vi "Software Update HCC Search For Archive.vi"(8 "error in (no error)":errorcluster, 10 "folder names":string[](array[string]), 11 "Path":path) -> (0 "error out":errorcluster, 3 "Output Path Archive Folder":path)   [LabVIEW 2016]
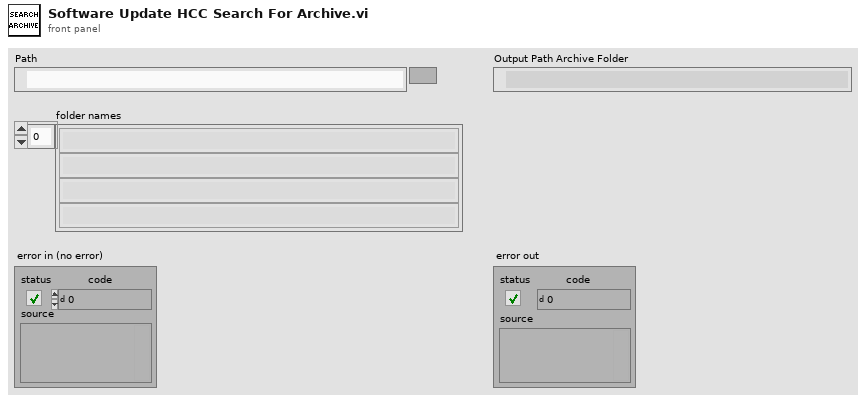
[diagram p1: front panel]
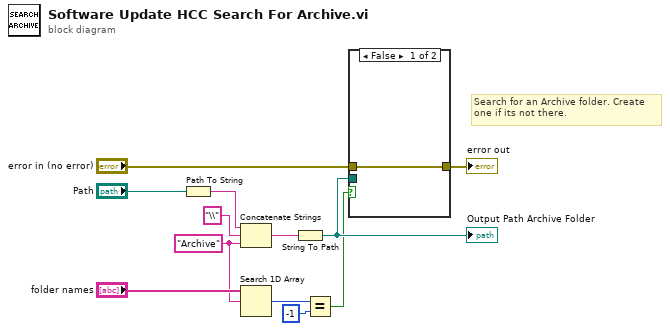
[diagram p0: block diagram]
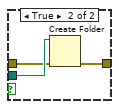
[diagram p2: hidden frame]
diagram:
  w2 = "Archive" ("element")
  # "Search for an Archive folder. Create\none if its not there."
  n1 = Path To String(path="Path") -> (string=w4:string)
  n2 = Concatenate Strings(w4, "\\" ("string"), w2) -> (w1:string)
  n3 = Search 1D Array(1D array="folder names", element=w2) -> (index of element=w7:i32)  [unwired: 1 in]
  n4 = String To Path(string=w1) -> (path=w10:path)
  "Output Path Archive Folder" <- w10
  n5 = Equal?(x=w7, y=-1) -> (x = y?=w5:bool)
  n6 = case shown="False" w5 {
    tunnel: w10 -> [_ w16]
    tunnel: "error in (no error)" -> [w13 w15]
    tunnel: [w13 w14] -> w9
    frame False {
    }
    frame True {
      n7 = Create Folder(path (use dialog)=w16, error in=w15) -> (error out=w14:errorcluster)  [unwired: 1 in, 2 out]
    }
  }
  "error out" <- w9
